vi "Main.vi"(10 "Messages Panel":refnum<vi>, 11 "Module Admin":refnum<class "Delacor_lib_QMH_Module Admin.lvclass">) -> ()   [LabVIEW 2019, in "MESSAGES.lvlib"]
doc: "This template is based off of the Queued Message Handler design pattern and the Queued Message Handler project template that ships with LabVIEW.\n\nThe main difference is that the queue is private to this module and communication between modules is performed via Broadcast and Request events.\n\nRequest events are wrapped in public API methods and are handled in the Event Handling Loop (EHL) of this VI. Any module can register for Broadcast events sent by this module. The EHL generates messages based on user interface actions.\n\nThe Message Handling Loop (MHL) processes messages generated by the EHL, or by other messages. The messages are string values, so new messages can be added easily to the Message Cases case structure in the MHL. Each message cluster can also provide an optional value for Message Data, which is a variant that can be converted to whatever message-specific data is required.\n_____\nBased on Delacor QMH Project Template 5.0.0.82."
uses:
  MESSAGES.lvlib
  <vilib>/Delacor/Delacor QMH/Libraries/Module Admin_class/Delacor_lib_QMH_Module Admin.lvclass
  Module Data--cluster.ctl
  Stop Argument--cluster.ctl
  <vilib>/Delacor/Delacor QMH/Libraries/Message Queue_class/Delacor_lib_QMH_Message Queue.lvclass/Delacor_lib_QMH_Message Queue.ctl
  <vilib>/Delacor/Delacor QMH/Libraries/Module Admin_class/Delacor_lib_QMH_Module Admin.lvclass/Delacor_lib_QMH_Module Admin.ctl
  SET MESSAGE Argument--cluster.ctl
  <vilib>/Utility/miscctls.llb/LVPointTypeDef.ctl
  <vilib>/Delacor/Delacor QMH/Libraries/Message Queue_class/Delacor_lib_QMH_Enqueue Message (Single).vi
  <vilib>/Delacor/Delacor QMH/Libraries/Module Admin_class/Delacor_lib_QMH_Get External Launch.vi
  <vilib>/Utility/error.llb/Error Cluster From Error Code.vi
  <vilib>/ErrorRing/Error Ring.xnode
  <vilib>/Delacor/Delacor QMH/Libraries/Message Queue_class/Delacor_lib_QMH_Message Queue.lvclass
panel:
  out "error out":errorcluster
  out "Status":string
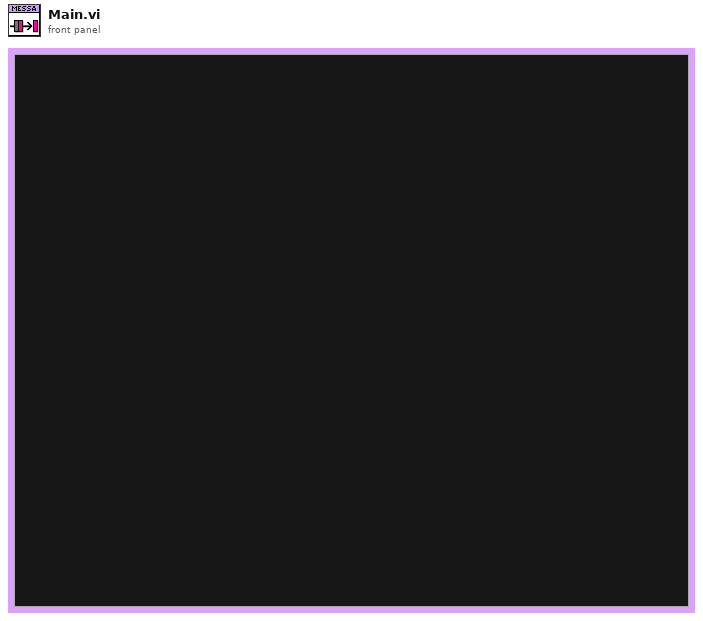
[diagram p1: front panel]
types:
  T1 = typedef "MESSAGES.lvlib/Request Events--cluster.ctl" = cluster{"Stop Module":refnum<user-event>, "Show Panel":refnum<user-event>, "Hide Panel":refnum<user-event>, "Get Module Execution Status":refnum<user-event>, "Show Diagram":refnum<user-event>, "SET MESSAGE":refnum<user-event>}
  T2 = typedef "MESSAGES.lvlib/Module Data--cluster.ctl" = cluster{"Status":string}
  T3 = enum32{"invalid lock state", "Not Locked", "Locked (No Password)", "Password-protected"}
  T4 = typedef "MESSAGES.lvlib/Stop Argument--cluster.ctl" = cluster{"Origin":string, "Exit via Stop Module Req?":bool, "Wait for Module to stop?":bool}
  T5 = typedef "MESSAGES.lvlib/SET MESSAGE Argument--cluster.ctl" = cluster{"Message":string}
  T6 = typedef "LVPointTypeDef.ctl" = cluster{"Horizontal":i16, "Vertical":i16}
  T7 = enum32{"Invalid", "Standard", "Closed", "Hidden", "Minimized", "Maximized"}
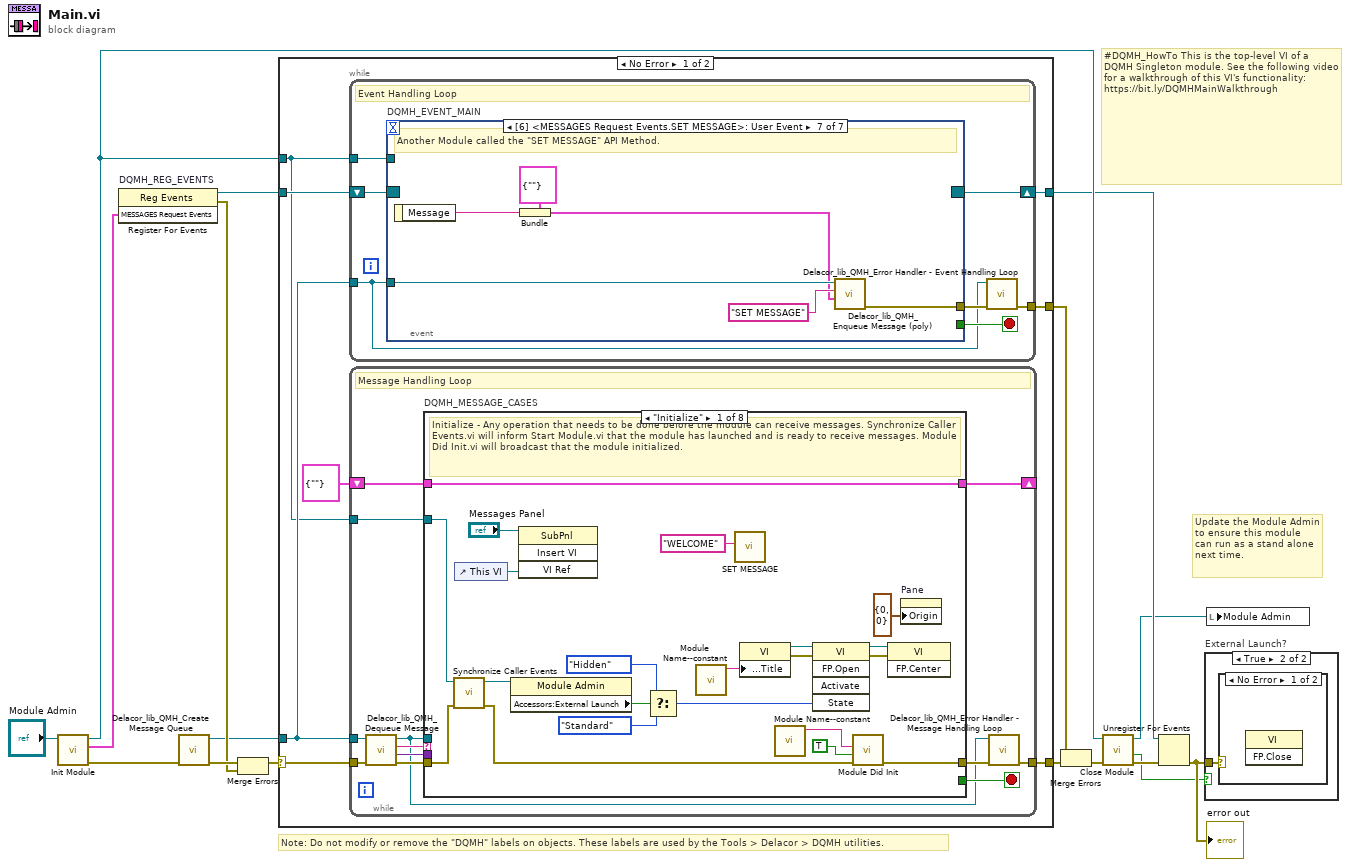
[diagram p0: block diagram]
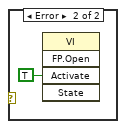
[diagram p3: hidden frame]
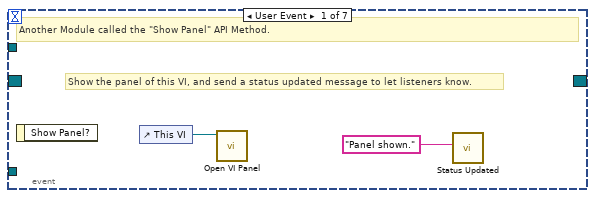
[diagram p4: hidden frame]
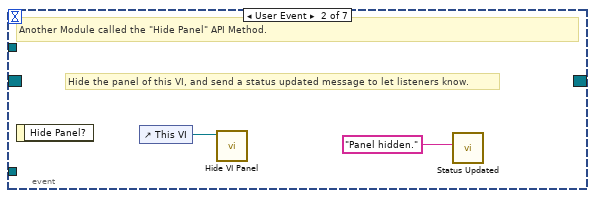
[diagram p5: hidden frame]
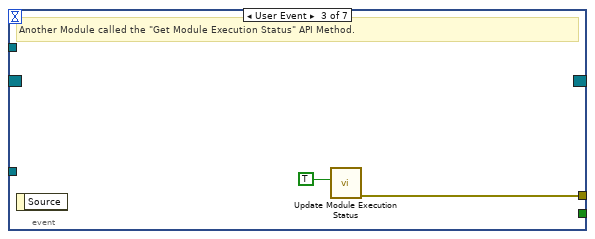
[diagram p6: hidden frame]
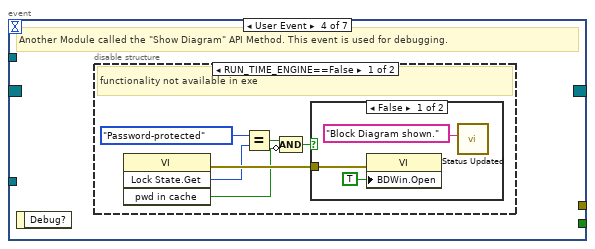
[diagram p7: hidden frame]
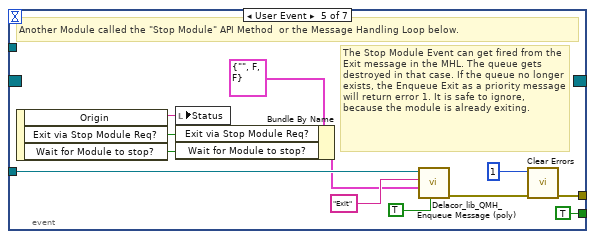
[diagram p10: hidden frame]
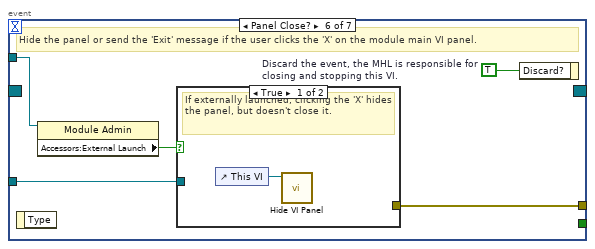
[diagram p11: hidden frame]
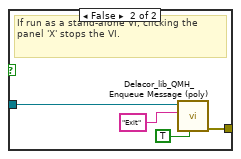
[diagram p12: hidden frame]
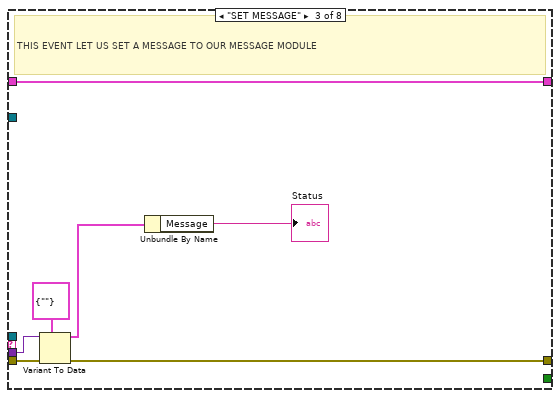
[diagram p14: hidden frame]
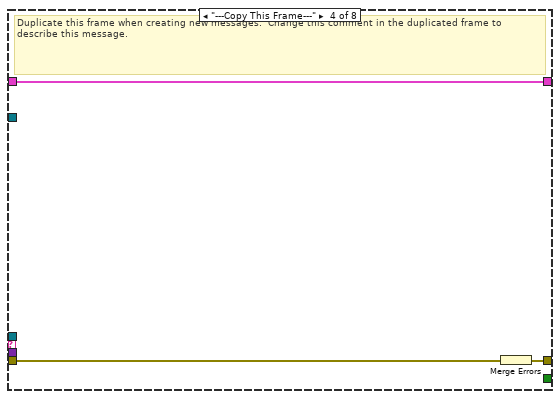
[diagram p15: hidden frame]
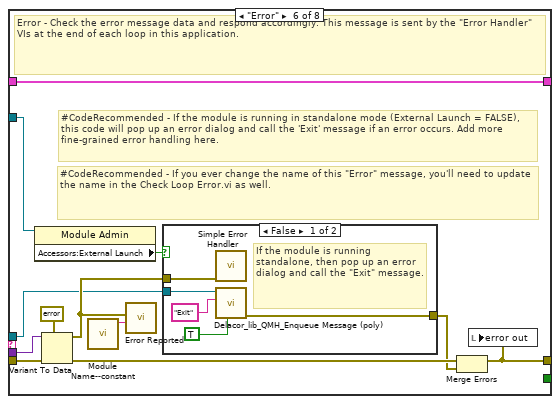
[diagram p17: hidden frame]
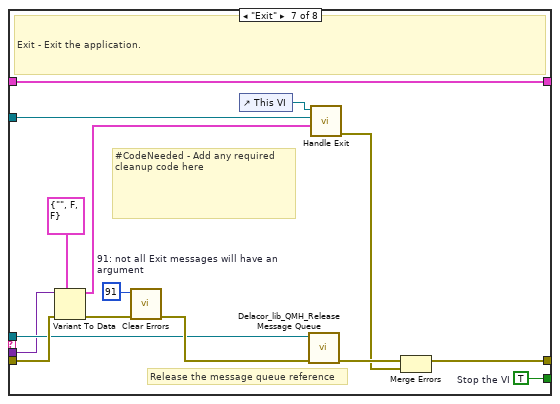
[diagram p19: hidden frame]
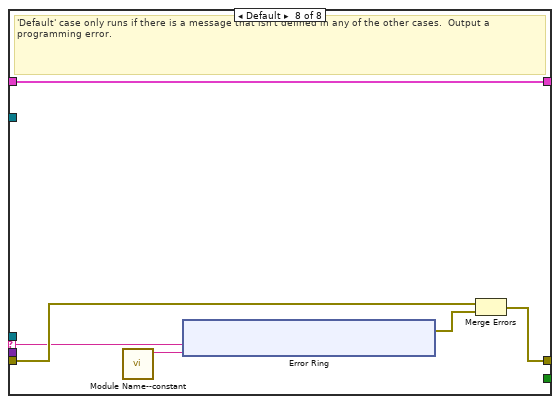
[diagram p20: hidden frame]
diagram:
  # "#DQMH_HowTo This is the top-level VI of a DQMH Singleton module. See the following video for a walkthrough of this VI's functionality: https://bit.ly/DQMHMainWalkthrough"
  # "Note: Do not modify or remove the \"DQMH\" labels on objects. These labels are used by the Tools > Delacor > DQMH utilities."
  # "Update the Module Admin to ensure this module can run as a stand alone next time."
  n1 = call "Init Module.vi"("Singleton Module Admin in"="Module Admin") -> ("error out"=w16:errorcluster, "MESSAGES Request Events"=w5:T1, "Singleton Module Admin out"=w8:refnum<class "Delacor_lib_QMH_Module Admin.lvclass">)  [unwired: 8 in]
  n2 = register-events "DQMH_REG_EVENTS"(w5) -> (reference out=w6:refnum<event-registration>, error out=w9:errorcluster)  [unwired: 2 in]
  n3 = call <vilib>:"Delacor_lib_QMH_Create Message Queue.vi"("error in (no error)"=w16) -> ("error out"=w11:errorcluster, "Message Queue"=w4:refnum<class "Delacor_lib_QMH_Message Queue.lvclass">)  [unwired: 9 in]
  n4 = Merge Errors(w11, w9) -> (w10:errorcluster)
  n5 = case shown="No Error" w10 {
    selector: w10 -> [w23 w171]
    tunnel: [w25 w170] -> w17
    tunnel: [w22 w176] -> w7
    tunnel: w6 -> [w20 w176]
    tunnel: w4 -> [w19 w169]
    tunnel: [w24 _] -> w14
    tunnel: w8 -> [w18 w172]
    frame No Error {
      n6 = while {
        tunnel: w19 -> [w26]
        shift-right: [w29] -> w22
        shift-left: w20 -> [w30]
        tunnel: [w31] -> w24
        tunnel: w18 -> [w27]
        stop <- w28 stop-if-true
        # "Event Handling Loop"
        n7 = event "DQMH_EVENT_MAIN" shown="[6] <MESSAGES Request Events.SET MESSAGE>: User Event" {
          selector: w30 -> [_ _ _ _ _ _ _]
          dyn-events: [_ _ _ _ _ _ _] -> w29
          timeout: _ -> [_ _ _ _ _ _ _]
          tunnel: [_ _ _ _ TRUE ("Discard?") _ _] -> w28
          tunnel: w26 -> [_ _ _ _ w55 w62 w75]
          tunnel: [_ _ w38 _ w58 w64 w70] -> w32
          tunnel: w27 -> [_ _ _ _ _ w61 _]
          event User Event {
            # "Show the panel of this VI, and send a status updated message to let listeners know."
            # "Another Module called the \"Show Panel\" API Method."
            n8 = event-data() -> ()  [unwired: 1 in, 1 out]
            n9 = control-ref of="This VI"() -> (w34:refnum<vi>)
            n10 = call "Open VI Panel.vi"("VI"=w34) -> ()  [unwired: 10 in, 1 out]
            n11 = call "Status Updated.vi"("Status"="Panel shown." ("format string")) -> ()  [unwired: 10 in, 1 out]
          }
          event User Event {
            # "Hide the panel of this VI, and send a status updated message to let listeners know."
            # "Another Module called the \"Hide Panel\" API Method."
            n12 = event-data() -> ()  [unwired: 1 in, 1 out]
            n13 = control-ref of="This VI"() -> (w36:refnum<vi>)
            n14 = call "Hide VI Panel.vi"("VI"=w36) -> ()  [unwired: 10 in, 1 out]
            n15 = call "Status Updated.vi"("Status"="Panel hidden." ("format string")) -> ()  [unwired: 10 in, 1 out]
          }
          event User Event {
            # "Another Module called the \"Get Module Execution Status\" API Method."
            n16 = event-data() -> ()  [unwired: 1 in, 1 out]
            n17 = call "Update Module Execution Status.vi"("Running?"=TRUE) -> ("error out"=w38:errorcluster)  [unwired: 10 in]
          }
          event User Event {
            # "Another Module called the \"Show Diagram\" API Method. This event is used for debugging."
            n18 = event-data() -> ()  [unwired: 1 in, 1 out]
            n19 = disable-structure shown="RUN_TIME_ENGINE==False" {
              frame condition #0 (active) {
                # "functionality not available in exe"
                n20 = invoke class="VI" method="Lock State.Get"() -> (error out=w44:errorcluster, "Get Lock State"=w43:T3, "pwd in cache"=w40:bool)  [unwired: 4 in, 1 out]
                n21 = Equal?(x=T3."Password-protected", y=w43) -> (x = y?=w41:bool)
                n22 = Compound Arithmetic op=AND(w41, invert w40) -> (w39:bool)
                n23 = case shown="False" w39 {
                  tunnel: w44 -> [w47 _]
                  frame False {
                    n24 = property class="VI"(error in=w47, "BDWin.Open"=TRUE ("Block Diagram Window:Open")) -> ()  [unwired: 1 in, 2 out]
                    n25 = call "Status Updated.vi"("Status"="Block Diagram shown." ("format string")) -> ()  [unwired: 10 in, 1 out]
                  }
                  frame True {
                    # "Password-protected VI, and the password is not in the cache. Do not show the diagram."
                  }
                }
              }
              frame condition #1 {
              }
            }
          }
          event User Event {
            # "The Stop Module Event can get fired from the Exit message in the MHL. The queue gets destroyed in that case. If the queue no longer exists, the Enqueue Exit as a priority message will return error 1. It is safe to ignore, because the module is already exiting."
            # "Another Module called the \"Stop Module\" API Method  or the Message Handling Loop below."
            n26 = event-data() -> ("Origin"=w54:string, "Exit via Stop Module Req?"=w50:bool, "Wait for Module to stop?"=w49:bool)  [unwired: 1 in]
            n27 = local write "Status"(w54) -> ()
            n28 = Bundle By Name(cluster=T4 {"Origin"="", "Exit via Stop Module Req?"=FALSE, "Wait for Module to stop?"=FALSE} ("Stop Argument"), "Exit via Stop Module Req?"=w50, "Wait for Module to stop?"=w49) -> (w48:T4)
            n29 = call-poly <vilib>:"Delacor_lib_QMH_Enqueue Message (poly).vi"("Priority Message? (F)"=TRUE, "Message Data"=w48, "Message"="Exit", "Message Queue in"=w55) -> ("error out"=w59:errorcluster)  [unwired: 6 in, 1 out]
            n30 = call <vilib>:"Clear Errors.vi"("error in (no error)"=w59, "specific error code to clear (0: all)"=1) -> ("error out"=w58:errorcluster)  [unwired: 4 in, 1 out]
          }
          event Panel Close? {
            w63 = TRUE  # Discard the event, the MHL is responsible for closing and stopping this VI.
            # "Hide the panel or send the 'Exit' message if the user clicks the 'X' on the module main VI panel."
            n31 = event-data() -> ()  [unwired: 1 in, 1 out]
            n32 = property class="Module Admin"(reference=w61) -> ("Accessors:External Launch"=w60:bool)  [unwired: 1 in, 2 out]
            n33 = case shown="True" w60 {
              tunnel: w62 -> [_ w68]
              tunnel: [_ w69] -> w64
              frame True {
                # "If externally launched, clicking the 'X' hides the panel, but doesn't close it."
                n34 = control-ref of="This VI"() -> (w65:refnum<vi>)
                n35 = call "Hide VI Panel.vi"("VI"=w65) -> ()  [unwired: 10 in, 1 out]
              }
              frame False {
                # "If run as a stand-alone VI, clicking the panel 'X' stops the VI."
                n36 = call-poly <vilib>:"Delacor_lib_QMH_Enqueue Message (poly).vi"("Priority Message? (F)"=TRUE, "Message"="Exit", "Message Queue in"=w68) -> ("error out"=w69:errorcluster)  [unwired: 7 in, 1 out]
              }
            }
            n37 = event-data("Discard?"=w63) -> ()  [unwired: 1 in, 1 out]
          }
          event User Event {
            # "Another Module called the \"SET MESSAGE\" API Method."
            n38 = event-data() -> ("Message"=w71:string)  [unwired: 1 in]
            n39 = Bundle(cluster=T5 {"Message"=""} ("SET MESSAGE Argument"), "Message"=w71) -> (w72:T5)
            n40 = call-poly <vilib>:"Delacor_lib_QMH_Enqueue Message (poly).vi"("Message Data"=w72, "Message"="SET MESSAGE", "Message Queue in"=w75) -> ("error out"=w70:errorcluster)  [unwired: 7 in, 1 out]
          }
        }
        n41 = call-dynamic "Delacor_lib_QMH_Error Handler - Event Handling Loop.vi"("error in (no error)"=w32, "Message Queue in"=w26) -> ("dup error in"=w31:errorcluster)  [unwired: 8 in, 1 out]
      }
      n42 = while {
        tunnel: w19 -> [w78]
        shift-right: [w82] -> _
        shift-left: T2 {"Status"=""} ("Data Cluster") -> [w83]
        tunnel: w23 -> [w86]
        tunnel: [w84] -> w25
        tunnel: w18 -> [w76]
        stop <- w81 stop-if-true
        # "Message Handling Loop"
        n43 = call-dynamic "Delacor_lib_QMH_Dequeue Message.vi"("error in (no error)"=w86, "Message Queue in"=w78) -> ("error out"=w85:errorcluster, "Message Data"=w79:variant, "Message"=w80:string, "Message Queue out"=w77:refnum<class "Delacor_lib_QMH_Message Queue.lvclass">)  [unwired: 6 in]
        n44 = case "DQMH_MESSAGE_CASES" shown="\"Initialize\"" w80 {
          selector: w80 -> [_ _ _ _ _ _ _ w156]
          tunnel: w77 -> [_ _ _ _ _ w126 w148 _]
          tunnel: w85 -> [w106 w110 w117 w120 w122 w133 w154 w158]
          tunnel: [w104 w110 w115 w119 w122 w129 w151 w159] -> w87
          tunnel: w83 -> [w95 w109 w116 w118 w121 w128 w147 w157]
          tunnel: [w95 w109 w116 w118 w121 w128 w147 w157] -> w82
          tunnel: [_ _ _ _ _ _ w146 _] -> w81
          tunnel: w79 -> [_ _ w114 _ _ w127 w145 _]
          tunnel: w76 -> [w96 _ _ _ _ w125 w140 _]
          frame "Initialize" {
            # "Initialize - Any operation that needs to be done before the module can receive messages. Synchronize Caller Events.vi will inform Start Module.vi that the module has launched and is ready to receive messages. Module Did Init.vi will broadcast that the module initialized."
            n45 = call "Synchronize Caller Events.vi"("error in (no error)"=w106, "Singleton Module Admin in"=w96) -> ("error out"=w105:errorcluster, "Singleton Module Admin out"=w92:refnum<class "Delacor_lib_QMH_Module Admin.lvclass">)  [unwired: 8 in]
            n46 = control-ref of="This VI"() -> (w89:refnum<vi>)
            n47 = property class="Module Admin"(reference=w92) -> ("Accessors:External Launch"=w100:bool)  [unwired: 1 in, 2 out]
            n48 = invoke class="SubPnl" method="Insert VI"(reference="Messages Panel", "VI Ref"=w89) -> ()  [unwired: 2 in, 4 out]
            n49 = Select(t=T7."Hidden" ("State"), s=w100, f=T7."Standard" ("State")) -> (s? t:f=w97:T7)
            n50 = call "Module Name--constant.vi"() -> ("Module Name"=w103:string)  [unwired: 11 in]
            n51 = call "SET MESSAGE.vi"("Message"="WELCOME") -> ()  [unwired: 10 in, 1 out]
            n52 = property class="VI"("Front Panel.Title"=w103) -> (reference out=w102:refnum<vi>, error out=w108:errorcluster)  [unwired: 2 in]
            n53 = call "Module Name--constant.vi"() -> ("Module Name"=w93:string)  [unwired: 11 in]
            n54 = invoke class="VI" method="FP.Open"(reference=w102, error in=w108, "State"=w97) -> (reference out=w101:refnum<vi>, error out=w107:errorcluster)  [unwired: 2 in, 3 out]
            n55 = call "Module Did Init.vi"("error in (no error)"=w105, "Initialized?"=TRUE, "Origin"=w93) -> ("error out"=w104:errorcluster)  [unwired: 8 in]
            n56 = invoke class="VI" method="FP.Center"(reference=w101, error in=w107) -> ()  [unwired: 1 in, 3 out]
            n57 = property on="Pane" class="Pane"("Origin"=T6 {"Horizontal"=0, "Vertical"=0}) -> ()  [unwired: 2 in, 2 out]
          }
          frame "--- Module Specific ---" {
            # "Separator -- The following cases handle messages specific to this Module."
          }
          frame "SET MESSAGE" {
            # "THIS EVENT LET US SET A MESSAGE TO OUR MESSAGE MODULE"
            n58 = Variant To Data(error in=w117, type=T5 {"Message"=""} ("SET MESSAGE Argument"), Variant=w114) -> (data=w112:T5, error out=w115:errorcluster)
            n59 = Unbundle By Name(w112) -> ("Message"=→"Status":string)
          }
          frame "---Copy This Frame---" {
            # "Duplicate this frame when creating new messages.  Change this comment in the duplicated frame to describe this message."
            n60 = Merge Errors(w120) -> (w119:errorcluster)
          }
          frame "--- Exit and Error Handling---" {
            # "Separator - The following cases handle errors and exit messages."
          }
          frame "Error" {
            # "#CodeRecommended - If you ever change the name of this \"Error\" message, you'll need to update the name in the Check Loop Error.vi as well."
            # "#CodeRecommended - If the module is running in standalone mode (External Launch = FALSE), this code will pop up an error dialog and call the 'Exit' message if an error occurs. Add more fine-grained error handling here."
            # "Error - Check the error message data and respond accordingly. This message is sent by the \"Error Handler\" VIs at the end of each loop in this application."
            n61 = property class="Module Admin"(reference=w125) -> ("Accessors:External Launch"=w124:bool)  [unwired: 1 in, 2 out]
            n62 = Variant To Data(error in=w133, type=errorcluster {"status"=FALSE, "code"=0, "source"=""} ("error constant"), Variant=w127) -> (data=w134:errorcluster, error out=w131:errorcluster)
            n63 = call "Module Name--constant.vi"() -> ("Module Name"=w123:string)  [unwired: 11 in]
            n64 = call "Error Reported.vi"("Additional Information"=w123, "Error"=w134) -> ()  [unwired: 9 in, 1 out]
            n65 = case shown="False" w124 {
              tunnel: [w139 _] -> w130
              tunnel: w126 -> [w137 _]
              tunnel: w134 -> [w138 _]
              frame False {
                # "If the module is running standalone, then pop up an error dialog and call the \"Exit\" message."
                n66 = call <vilib>:"Simple Error Handler.vi"("error in (no error)"=w138) -> ()  [unwired: 4 in, 5 out]
                n67 = call-poly <vilib>:"Delacor_lib_QMH_Enqueue Message (poly).vi"("Priority Message? (F)"=TRUE, "Message"="Exit", "Message Queue in"=w137) -> ("error out"=w139:errorcluster)  [unwired: 7 in, 1 out]
              }
              frame True {
                # "If the module was launched externally, calling the Error Reported broadcast VI is the only action performed by the \"Error\" message. The module's caller can then process the error appropriately."
              }
            }
            n68 = Merge Errors(w131, w130) -> (w129:errorcluster)
            n69 = local write "error out"(w129) -> ()
          }
          frame "Exit" {
            w144 = 91  # 91: not all Exit messages will have an argument
            w146 = TRUE  # Stop the VI
            # "Release the message queue reference"
            # "#CodeNeeded - Add any required cleanup code here"
            # "Exit - Exit the application."
            n70 = Variant To Data(error in=w154, type=T4 {"Origin"="", "Exit via Stop Module Req?"=FALSE, "Wait for Module to stop?"=FALSE} ("Stop Argument"), Variant=w145) -> (data=w142:T4, error out=w150:errorcluster)
            n71 = call <vilib>:"Clear Errors.vi"("error in (no error)"=w150, "specific error code to clear (0: all)"=w144) -> ("error out"=w153:errorcluster)  [unwired: 4 in, 1 out]
            n72 = control-ref of="This VI"() -> (w141:refnum<vi>)
            n73 = call-dynamic "Delacor_lib_QMH_Release Message Queue.vi"("error in (no error)"=w153, "Message Queue"=w148) -> ("error out"=w152:errorcluster)  [unwired: 9 in]
            n74 = call "Handle Exit.vi"("Stop Argument"=w142, "Admin in"=w140, "VI reference"=w141) -> ("error out"=w149:errorcluster)  [unwired: 7 in, 1 out]
            n75 = Merge Errors(w152, w149) -> (w151:errorcluster)
          }
          frame Default {
            # "'Default' case only runs if there is a message that isn't defined in any of the other cases.  Output a programming error."
            n76 = call "Module Name--constant.vi"() -> ("Module Name"=w155:string)  [unwired: 11 in]
            n77 = xnode "Error Ring"("parameter 0"=w156, "parameter 1"=w155) -> ("error out"=w160:errorcluster)
            n78 = Merge Errors(w158, w160) -> (w159:errorcluster)
          }
        }
        n79 = call-dynamic "Delacor_lib_QMH_Error Handler - Message Handling Loop.vi"("error in (no error)"=w87, "Message Queue in"=w77) -> ("dup error in"=w84:errorcluster)  [unwired: 8 in, 1 out]
      }
    }
    frame Error {
      # "Synchronize Caller Events.vi will inform Start Module.vi that the module has launched and will let the code calling Start Module.vi register for broadcasts and would permit the caller receive the broadcast that an error occurred at launch time."
      n80 = call-dynamic "Delacor_lib_QMH_Release Message Queue.vi"("error in (no error)"=w171, "Message Queue"=w169) -> ("error out"=w170:errorcluster)  [unwired: 9 in]
      n81 = call "Synchronize Caller Events.vi"("Singleton Module Admin in"=w172) -> ("error out"=w177:errorcluster)  [unwired: 9 in, 1 out]
      n82 = call "Module Name--constant.vi"() -> ("Module Name"=w175:string)  [unwired: 11 in]
      n83 = Format Into String(format string="An error occurred during initialization. %s is no longer running.", w175) -> (resulting string=w173:string)  [unwired: 2 in, 1 out]
      n84 = Merge Errors(w170, w177) -> (w178:errorcluster)
      n85 = call "Error Reported.vi"("Additional Information"=w173, "Error"=w178) -> ()  [unwired: 9 in, 1 out]
    }
  }
  n86 = Merge Errors(w14, w17) -> (w13:errorcluster)
  n87 = call "Close Module.vi"("error in (no error)"=w13, "Module Admin in"=w8) -> ("error out"=w15:errorcluster, "External Launch"=w1:bool, "Module Admin out"=w2:refnum<class "Delacor_lib_QMH_Module Admin.lvclass">)  [unwired: 7 in]
  n88 = Unregister For Events(event registration refnum=w7, error in=w15) -> (error out=w12:errorcluster)
  "error out" <- w12
  n89 = case "External Launch?" shown="True" w1 {
    tunnel: w12 -> [_ w179]
    frame False {
    }
    frame True {
      n90 = case shown="No Error" w179 {
        frame No Error {
          n91 = invoke class="VI" method="FP.Close"() -> ()  [unwired: 3 in, 3 out]
        }
        frame Error {
          n92 = invoke class="VI" method="FP.Open"("Activate"=TRUE ("Activate?")) -> ()  [unwired: 4 in, 5 out]
        }
      }
    }
  }
  n93 = local write "Module Admin"(w2) -> ()
